vi "ConfigMultifileWrite.vi"(10 "Reference":T1) -> (2 "Data Valid":bool)   [LabVIEW 2017]
uses:
  <vilib>/express/express shared/propPageData.ctl
panel:
  in  "max_elapsed_seconds":i32
  in  "Time":i32 min=0 max=86399 step=60 format="%<%H:%M>t"
  in  "Hours":i32 min=0 max=999
  in  "Help":bool
  in  "Ok":bool
  in  "Cancel":bool
  in  "overwrite_mode_multi":i32
  in  "new_file_mode":i32
  in  "Use next available filename":bool
  in  "Overwrite file":bool
  in  "Rename existing file":bool
  out "Filename preview":string
  in  "Both":bool
  in  "fixed_width":bool=TRUE
  in  "Width":i32=2 min=1 max=9
  in  "Date and time":bool=TRUE
  in  "Sequential numbers":bool
  in  "Samples":i32=1 min=1
  in  "Segments":i32=1 min=1
  in  "new_file_samples":bool
  in  "new_file_iter":bool
  in  "new_file_daily":bool
  in  "Minutes":i32 min=0 max=59
  in  "new_file_elaps_time":bool
  in  "KB":i32=100
  in  "new_file_size":bool=TRUE
  in  "file_path":path=path "testdata_.txt"
  in  "time_format_string":string="%Y-%m-%d"
  # "Filename Suffix"
  # "File Termination"
  # "Condition for starting a new file"
  # "Existing Files"
  # "Action to take if the file already exists"
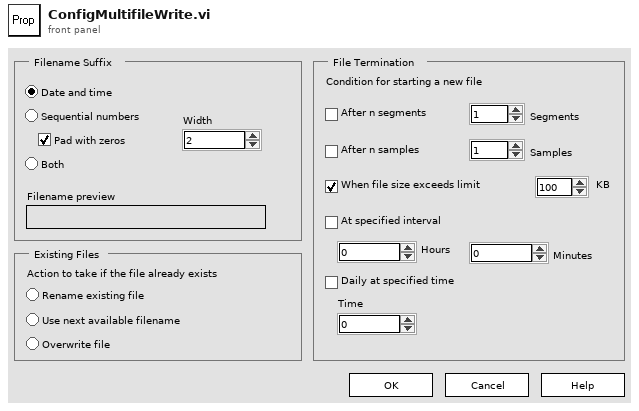
[diagram p1: front panel]
types:
  T1 = typedef "propPageData.ctl" = cluster{"InstanceCtlRefs":refnum<vi>[], "ConfigDlgCtlRefs":refnum<vi>[], "Control Data":cluster{"Ctl Type":u16, "Instance Ctl Label":string, "Config Dialog Ctl Label":string}[], "viref Instance":refnum<vi>, "Types":i32[], "Config DialogVI":refnum<vi>}
  T2 = enum8{"Enabled", "Disabled", "Disabled and Grayed Out"}
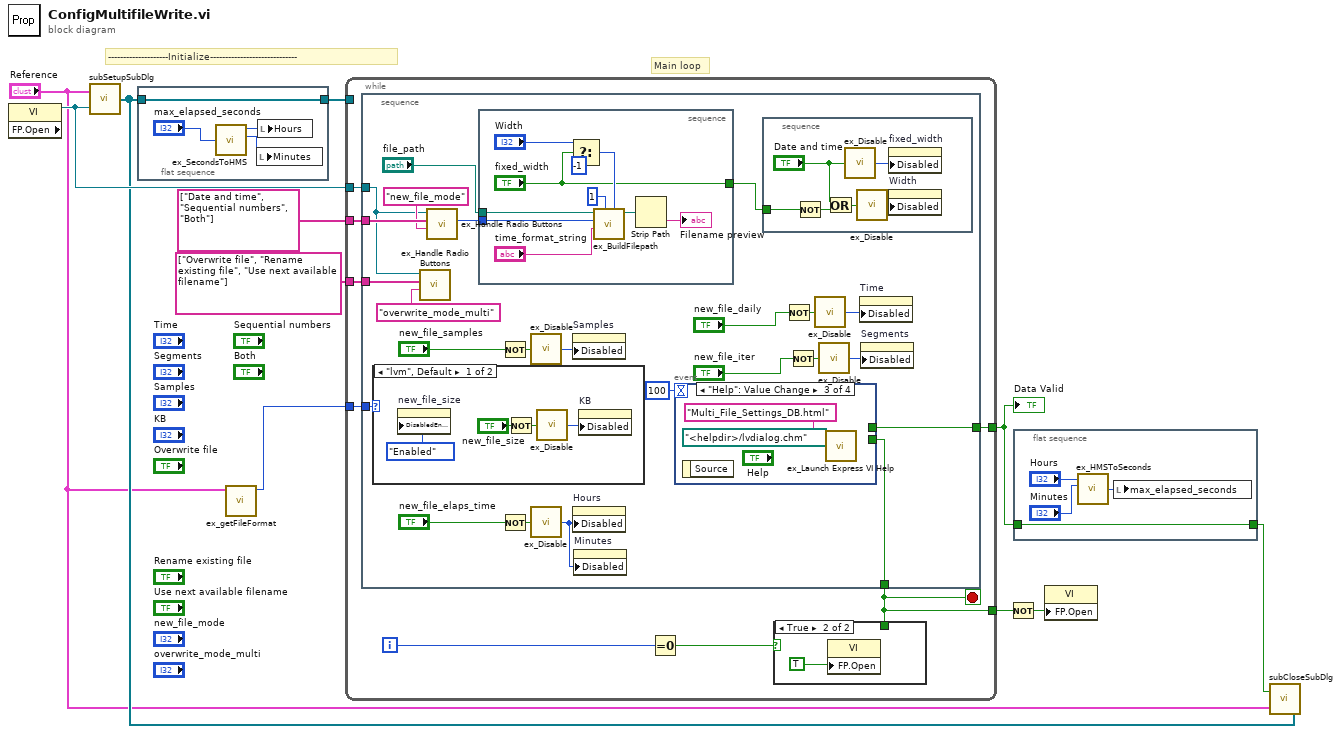
[diagram p0: block diagram]
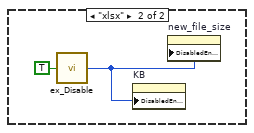
[diagram p3: hidden frame]
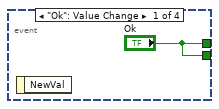
[diagram p4: hidden frame]
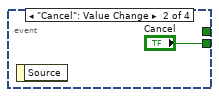
[diagram p5: hidden frame]
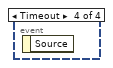
[diagram p6: hidden frame]
diagram:
  # "--------------------Initialize-----------------------------"
  # "Main loop"
  n1 = property class="VI" props=["FP.Open"]() -> (reference out=w10:refnum<vi>)  [unwired: 2 in, 2 out]
  n2 = call <vilib>:"subSetupSubDlg.vi"("viref subdlg"=w10, "Reference"="Reference") -> ("subDlgRefs"=w8:refnum<vi>[])
  n3 = flat-sequence {
    tunnel: w8 -> [w13]
    tunnel: [w13] -> w7
    frame #0 {
      n4 = call <vilib>:"ex_SecondsToHMS.vi"("seconds"="max_elapsed_seconds") -> ("hours"=w14:i32, "minutes"=w12:i32)  [unwired: 2 out]
      n5 = local write "Minutes"(w12) -> ()
      n6 = local write "Hours"(w14) -> ()
    }
  }
  n7 = call <vilib>:"ex_getFileFormat.vi"("Reference"="Reference") -> ("storage_format"=w1:enum32{"lvm", "tdm", "tdms", "xlsx"})  [unwired: 10 in]
  n8 = while {
    tunnel: [w23] -> w6
    tunnel: w10 -> [w21]
    tunnel: string[] ["Date and time", "Sequential numbers", "Both"] ("Radio Buttons") -> [w22]
    tunnel: string[] ["Overwrite file", "Rename existing file", "Use next available filename"] ("Radio Buttons") -> [w20]
    tunnel: w7 -> [_]
    tunnel: [w17] -> w3
    tunnel: w1 -> [w16]
    i -> [w18]
    stop <- w17 stop-if-true
    n9 = stacked-sequence {
      tunnel: [w32] -> w23
      tunnel: w22 -> [w48]
      tunnel: w21 -> [w36]
      tunnel: [w31] -> w17
      tunnel: w20 -> [w38]
      tunnel: w16 -> [w25]
      frame #0 {
        n10 = case shown="\"lvm\", Default" w25 {
          frame "lvm", Default {
            n11 = property on="new_file_size" class="Bool (strict)"("DisabledEnum"=T2."Enabled" ("Disabled")) -> ()  [unwired: 2 in, 2 out]
            n12 = Not(x="new_file_size") -> (.not. x?=w50:bool)
            n13 = call <vilib>:"ex_Disable.vi"("Disable?"=w50) -> ("Disabled value"=w51:u8)
            n14 = property on="KB" class="DigNum (strict)"("Disabled"=w51) -> ()  [unwired: 2 in, 2 out]
          }
          frame "xlsx" {
            n15 = call <vilib>:"ex_Disable.vi"("Disable?"=TRUE) -> ("Disabled value"=w53:u8)
            n16 = property on="KB" class="DigNum (strict)"("DisabledEnum"=w53) -> ()  [unwired: 2 in, 2 out]
            n17 = property on="new_file_size" class="Bool (strict)"("DisabledEnum"=w53) -> ()  [unwired: 2 in, 2 out]
          }
        }
        n18 = call <vilib>:"ex_Handle Radio Buttons.vi"("Numeric Control"="overwrite_mode_multi", "Radio Buttons"=w38, "VI refnum"=w36) -> ()  [unwired: 4 in, 5 out]
        n19 = call <vilib>:"ex_Handle Radio Buttons.vi"("Numeric Control"="new_file_mode", "Radio Buttons"=w48, "VI refnum"=w36) -> ("Selected Button"=w35:u32)  [unwired: 4 in, 4 out]
        n20 = stacked-sequence {
          tunnel: w35 -> [w74]
          tunnel: "file_path" -> [w70]
          tunnel: ["fixed_width"] -> w40
          frame #0 {
            n21 = Select(t="Width", s="fixed_width", f=-1 ("serno_digits")) -> (s? t:f=w72:i32)
            n22 = call <vilib>:"ex_BuildFilepath.vi"("serial digits"=w72, "serial num"=1, "time format string"="time_format_string", "naming mode"=w74, "name base"=w70) -> ("built name"=w69:path)  [unwired: 1 in, 5 out]
            n23 = Strip Path(path=w69) -> (name=→"Filename preview":string)  [unwired: 1 out]
          }
        }
        n24 = Not(x="new_file_samples") -> (.not. x?=w42:bool)
        n25 = Not(x="new_file_elaps_time") -> (.not. x?=w47:bool)
        n26 = call <vilib>:"ex_Disable.vi"("Disable?"=w42) -> ("Disabled value"=w41:u8)
        n27 = call <vilib>:"ex_Disable.vi"("Disable?"=w47) -> ("Disabled value"=w46:u8)
        n28 = property on="Samples" class="DigNum (strict)"("Disabled"=w41) -> ()  [unwired: 2 in, 2 out]
        n29 = property on="Hours" class="DigNum (strict)"("Disabled"=w46) -> ()  [unwired: 2 in, 2 out]
        n30 = property on="Minutes" class="DigNum (strict)"("Disabled"=w46) -> ()  [unwired: 2 in, 2 out]
        n31 = event shown="[2] \"Help\": Value Change" {
          selector: _ -> [_ _ _ _]
          dyn-events: _ -> [_ _ _ _]
          timeout: 100 -> [_ _ _ _]
          tunnel: ["Ok" _ _ _] -> w32
          tunnel: ["Ok" "Cancel" _ _] -> w31
          event "Ok": Value Change {
            n32 = event-data() -> ()  [unwired: 2 out]
          }
          event "Cancel": Value Change {
            n33 = event-data() -> ()  [unwired: 2 out]
          }
          event "Help": Value Change {
            n34 = event-data() -> ()  [unwired: 2 out]
            n35 = call <vilib>:"ex_Launch Express VI Help.vi"("Help File Path"=path "<helpdir>/lvdialog.chm", "Keyword/HTML File"="Multi_File_Settings_DB.html" ("Help string to search for")) -> ()  [unwired: 1 in, 5 out]
          }
          event Timeout {
            n36 = event-data() -> ()  [unwired: 2 out]
          }
        }
        n37 = stacked-sequence {
          tunnel: w40 -> [w64]
          frame #0 {
            n38 = Not(x=w64) -> (.not. x?=w60:bool)
            n39 = Or(x="Date and time", y=w60) -> (x .or. y?=w61:bool)
            n40 = call <vilib>:"ex_Disable.vi"("Disable?"="Date and time") -> ("Disabled value"=w63:u8)
            n41 = call <vilib>:"ex_Disable.vi"("Disable?"=w61) -> ("Disabled value"=w62:u8)
            n42 = property on="fixed_width" class="Bool (strict)"("Disabled"=w63) -> ()  [unwired: 2 in, 2 out]
            n43 = property on="Width" class="DigNum (strict)"("Disabled"=w62) -> ()  [unwired: 2 in, 2 out]
          }
        }
        n44 = Not(x="new_file_daily") -> (.not. x?=w45:bool)
        n45 = Not(x="new_file_iter") -> (.not. x?=w44:bool)
        n46 = call <vilib>:"ex_Disable.vi"("Disable?"=w45) -> ("Disabled value"=w33:u8)
        n47 = call <vilib>:"ex_Disable.vi"("Disable?"=w44) -> ("Disabled value"=w43:u8)
        n48 = property on="Time" class="DigNum (strict)"("Disabled"=w33) -> ()  [unwired: 2 in, 2 out]
        n49 = property on="Segments" class="DigNum (strict)"("Disabled"=w43) -> ()  [unwired: 2 in, 2 out]
      }
    }
    n50 = Equal To 0?(x=w18) -> (x = 0?=w19:bool)
    n51 = case shown="True" w19 {
      tunnel: w17 -> [_ _]
      frame False {
      }
      frame True {
        n52 = property class="VI"("FP.Open"=TRUE ("Front Panel Window:Open")) -> ()  [unwired: 2 in, 2 out]
      }
    }
  }
  "Data Valid" <- w6
  n53 = Not(x=w3) -> (.not. x?=w4:bool)
  n54 = flat-sequence {
    tunnel: w6 -> [w78]
    tunnel: [w78] -> w5
    frame #0 {
      n55 = call <vilib>:"ex_HMSToSeconds.vi"("minutes"="Minutes", "hours"="Hours") -> ("seconds"=w75:i32)  [unwired: 1 in, 1 out]
      n56 = local write "max_elapsed_seconds"(w75) -> ()
    }
  }
  n57 = property class="VI"("FP.Open"=w4) -> ()  [unwired: 2 in, 2 out]
  n58 = call <vilib>:"subCloseSubDlg.vi"("subDlgRefs"=w8, "Reference"="Reference", "OK Pressed"=w5) -> ()
